vi "Test Simple Request.vi"(11 "Test Case In":refnum<class "Test Commands.lvclass">) -> (0 "error out":errorcluster, 3 "Test Case Out":refnum<class "Test Commands.lvclass">)   [LabVIEW 2019, in "Test Commands.lvclass"]
uses:
  Test Commands.lvclass
  C:/Program Files (x86)/National Instruments/LabVIEW 2024/vi.lib/Astemes/LUnit/Test Case.lvclass
  Test Commands.lvclass/Test Commands.ctl
  <vilib>/Astemes/LUnit/Test Case.lvclass/Test Case.ctl
  <vilib>/Astemes/LUnit/Core/LUnit Test Case/Private/Append Fail Result.vi
  <vilib>/Astemes/LUnit/Core/LUnit Test Case/Private/Append Pass Result.vi
  <vilib>/Astemes/LUnit/Core/LUnit Test Case/Private/Run In UI.vi
  <vilib>/Utility/error.llb/Clear Errors.vi
  <vilib>/Astemes/LUnit/Test Case.lvclass
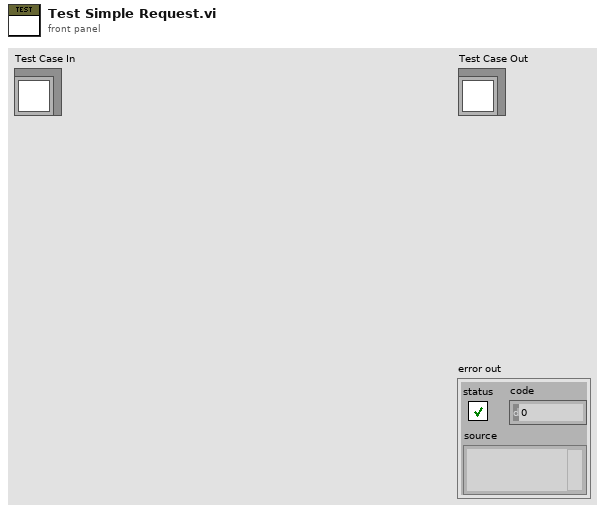
[diagram p1: front panel]
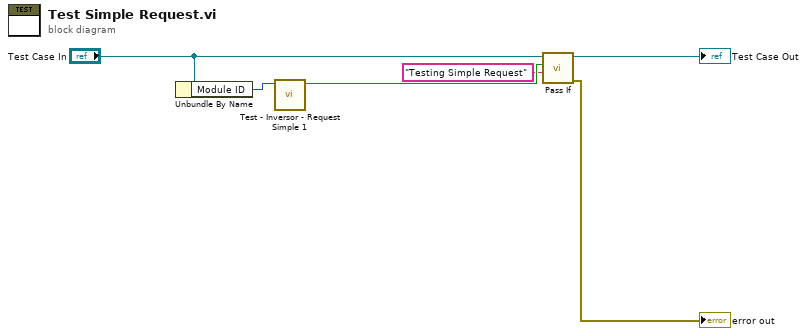
[diagram p0: block diagram]
diagram:
  n1 = Unbundle By Name("Test Case In") -> ("Module ID"=w3:i32)
  n2 = call "Test - Inversor - Request Simple 1.vi"("Module ID"=w3) -> ("Pass"=w2:bool)  [unwired: 9 in, 1 out]
  n3 = call <vilib>:"Pass If.vi"("Message"="Testing Simple Request", "Pass?"=w2, "LUnit Test Case In"="Test Case In") -> ("error out"=→"error out":errorcluster, "LUnit Test Case Out"=→"Test Case Out":refnum<class "Test Commands.lvclass">)  [unwired: 7 in]
